vi "CaseStatement.vi"() -> ()   [LabVIEW 2014]
panel:
  in  "Operation":bool
  out "Result":dbl
  in  "B":dbl
  in  "A":dbl
  out "Multiplied":bool
  # "Multiply"
  # "Add"
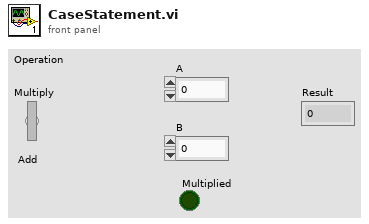
[diagram p1: front panel]
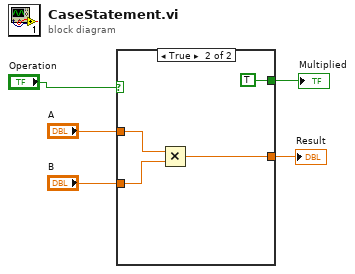
[diagram p0: block diagram]
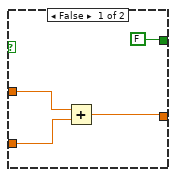
[diagram p2: hidden frame]
diagram:
  n1 = case shown="True" "Operation" {
    tunnel: "A" -> [w9 w13]
    tunnel: "B" -> [w8 w12]
    tunnel: [w7 w11] -> w3
    tunnel: [FALSE TRUE] -> w2
    frame False {
      n2 = Add(x=w9, y=w8) -> (x+y=w7:dbl)
    }
    frame True {
      n3 = Multiply(x=w13, y=w12) -> (x*y=w11:dbl)
    }
  }
  "Multiplied" <- w2
  "Result" <- w3
